vi "Module Loop.vi"(8 "error in (no error)":errorcluster, 11 "SoftVar Module in":refnum<class "SoftVar Module.lvclass">) -> (0 "error out":errorcluster, 3 "SoftVar Module out":refnum<class "SoftVar Module.lvclass">)   [LabVIEW 2023, in "Volatus.lvlib" / "SoftVar Module.lvclass"]
uses:
  SoftVar Module.lvclass
  SoftVar Module.lvclass/SoftVar Module.ctl
  Module/Module.lvclass
  messages/CmdAnalog/Data.ctl
  messages/CmdAnalog/CmdAnalog.lvlib
  lv-vecto/Vecto/Vecto.lvlib
  lv-vecto/Vecto/Group DBL/Group DBL.lvclass
  C:/dev/volatus/mts-volatus-super/libs/lv-volatus/Volatus/Module/Module.lvclass
  C:/dev/volatus/mts-volatus-super/libs/lv-volatus/Volatus/SoftVar Module/SoftVar Module.lvclass
panel:
  in  "Display":bool
  out "Values":T1(array[cluster])
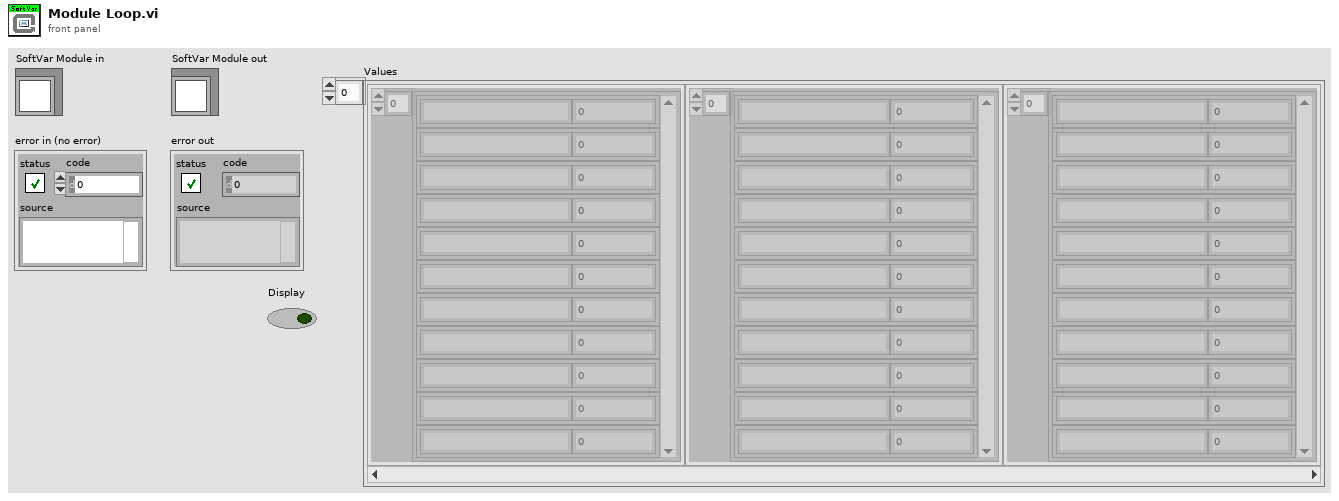
[diagram p1: front panel]
types:
  T1 = cluster{cluster{"Name":string, "Scaled":dbl}[]}[]
  T2 = enum32{"Invalid", "Standard", "Closed", "Hidden", "Minimized", "Maximized"}
  T3 = typedef "CmdAnalog.lvlib/Data.ctl" = cluster{"channel":string, "value":dbl}
  T4 = cluster{cluster{"String":string, "Scaled":dbl}[]}
  T5 = typedef "CmdAnalogMultiple.lvlib/Data.ctl" = cluster{"values":T3[]}
  T6 = typedef "CmdDigitalMultiple.lvlib/Data.ctl" = cluster{"values":T7[]}
  T7 = typedef "CmdDigital.lvlib/Data.ctl" = cluster{"channel":string, "value":bool}
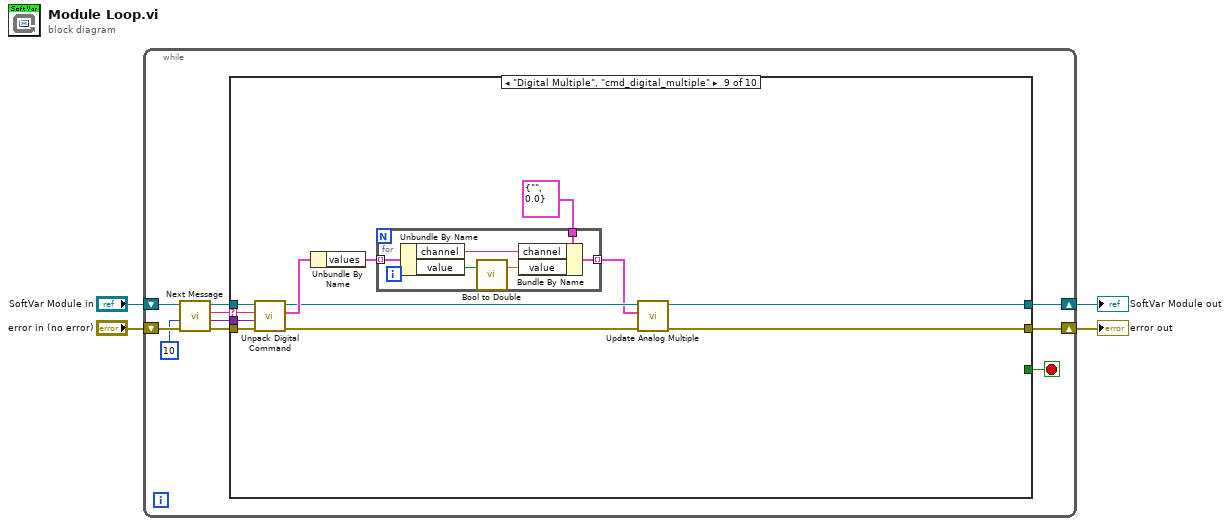
[diagram p0: block diagram]
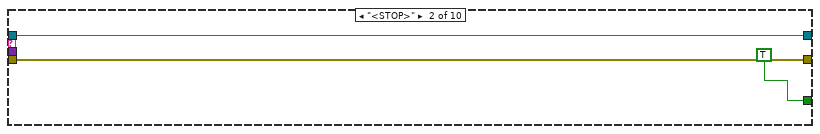
[diagram p3: hidden frame]
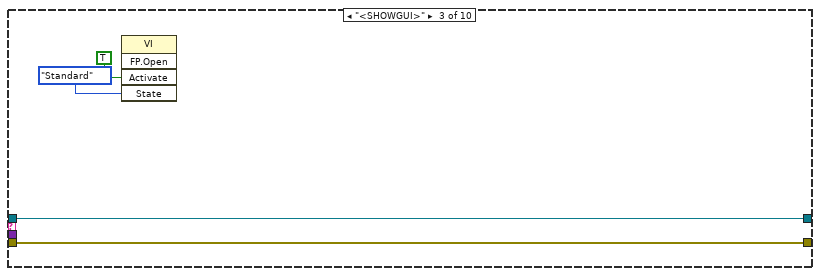
[diagram p4: hidden frame]
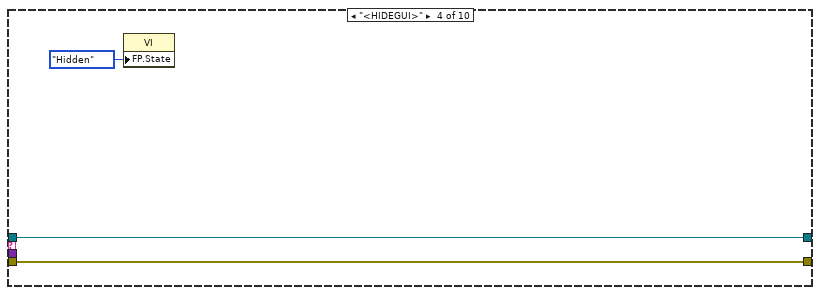
[diagram p5: hidden frame]
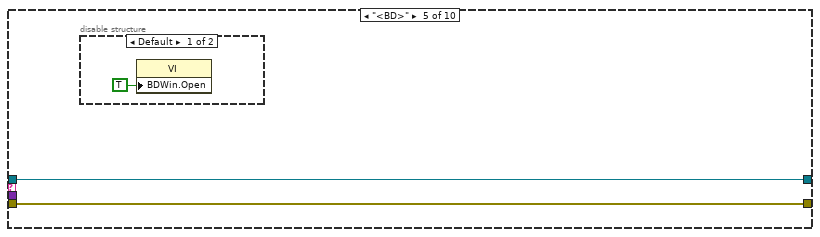
[diagram p6: hidden frame]
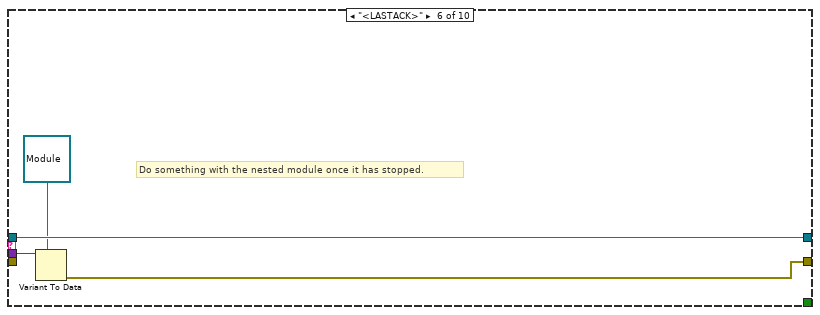
[diagram p8: hidden frame]
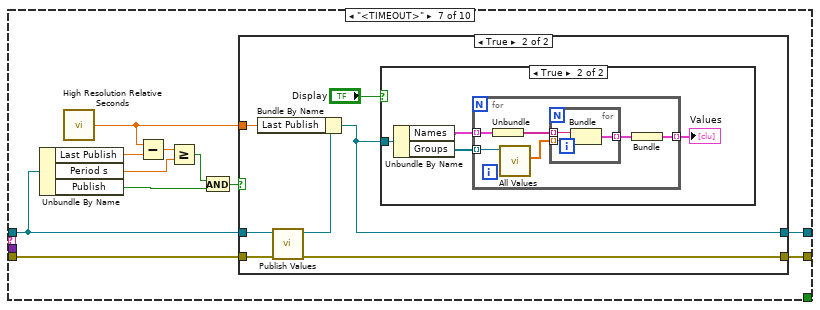
[diagram p9: hidden frame]
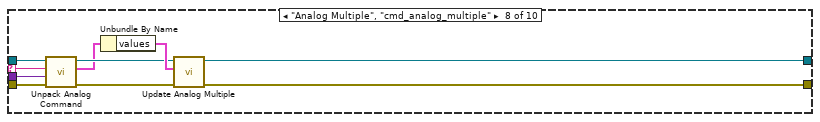
[diagram p12: hidden frame]
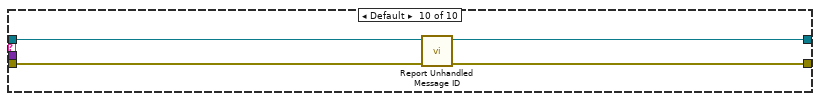
[diagram p13: hidden frame]
diagram:
  n1 = while {
    shift-right: [w9] -> w2
    shift-left: "SoftVar Module in" -> [w14]
    shift-right: [w8] -> w1
    shift-left: "error in (no error)" -> [w13]
    stop <- w7 stop-if-true
    n2 = call "Next Message.vi"("error in (no error)"=w13, "Timeout/Period ms (-1)"=10 ("Timeout ms (-1)"), "Module in"=w14) -> ("error out"=w12:errorcluster, "Data"=w6:variant, "ID"=w11:string, "Module out"=w10:refnum<class "SoftVar Module.lvclass">)  [unwired: 5 in]
    n3 = case shown="\"Digital Multiple\", \"cmd_digital_multiple\"" w11 {
      selector: w11 -> [_ _ _ _ _ _ _ w72 w84 _]
      tunnel: w12 -> [w15 w18 w22 w25 w27 _ w41 w70 w85 w98]
      tunnel: w10 -> [w16 w19 w23 w26 w28 w33 w42 w73 w86 w96]
      tunnel: [w16 w19 w23 w26 w28 w33 w34 w74 w78 w95] -> w9
      tunnel: [w15 w18 w22 w25 w27 w30 w35 w75 w77 w97] -> w8
      tunnel: [_ TRUE _ _ _ _ _ _ _ _] -> w7
      tunnel: w6 -> [_ _ _ _ _ w32 _ w71 w83 _]
      frame "<CLOSE>" {
      }
      frame "<STOP>" {
      }
      frame "<SHOWGUI>" {
        n4 = invoke class="VI" method="FP.Open"("Activate"=TRUE ("Activate?"), "State"=T2."Standard") -> ()  [unwired: 3 in, 5 out]
      }
      frame "<HIDEGUI>" {
        n5 = property class="VI"("FP.State"=T2."Hidden" ("Front Panel Window:State")) -> ()  [unwired: 2 in, 2 out]
      }
      frame "<BD>" {
        n6 = disable-structure shown="Default" {
          frame condition #0 (active) {
            n7 = property class="VI"("BDWin.Open"=TRUE ("Block Diagram Window:Open")) -> ()  [unwired: 2 in, 2 out]
          }
          frame condition #1 {
          }
        }
      }
      frame "<LASTACK>" {
        # "Do something with the nested module once it has stopped."
        n8 = Variant To Data(type=refnum<class "Module.lvclass"> refnum ("Volatus:Module"), Variant=w32) -> (error out=w30:errorcluster)  [unwired: 1 in, 1 out]
      }
      frame "<TIMEOUT>" {
        n9 = Unbundle By Name(w42) -> ("Last Publish"=w44:dbl, "Period s"=w38:dbl, "Publish"=w39:bool)
        n10 = call <vilib>:"High Resolution Relative Seconds.vi"() -> ("relative seconds"=w36:dbl)
        n11 = Subtract(x=w36, y=w44) -> (x-y=w43:dbl)
        n12 = Greater Or Equal?(x=w43, y=w38) -> (x >= y?=w40:bool)
        n13 = And(x=w40, y=w39) -> (x .and. y?=w37:bool)
        n14 = case shown="True" w37 {
          tunnel: w42 -> [w46 w53]
          tunnel: w41 -> [w45 w52]
          tunnel: w36 -> [_ w50]
          tunnel: [w45 w49] -> w35
          tunnel: [w46 w48] -> w34
          frame False {
          }
          frame True {
            n15 = call "Publish Values.vi"("error in (no error)"=w52, "SoftVar Module in"=w53) -> ("error out"=w49:errorcluster, "SoftVar Module out"=w51:refnum<class "SoftVar Module.lvclass">)  [unwired: 8 in]
            n16 = Bundle By Name(cluster=w51, "Last Publish"=w50) -> (w48:refnum<class "SoftVar Module.lvclass">)
            n17 = case shown="True" "Display" {
              tunnel: w48 -> [_ w57]
              frame False {
              }
              frame True {
                n18 = Unbundle By Name(w57) -> ("Names"=w54:cluster{"Names":string[]}[], "Groups"=w56:refnum<class "Group DBL.lvclass">[])
                n19 = for {
                  tunnel: w56 -> [w60] mode=indexing
                  tunnel: [w61] -> w55 mode=indexing
                  tunnel: w54 -> [w59] mode=indexing
                  n20 = Unbundle(w59) -> ("Names"=w58:string[])
                  n21 = call "All Values.vi"("Group in"=w60) -> ("Scaled"=w63:dbl[])  [unwired: 6 in, 4 out]
                  n22 = for {
                    tunnel: w58 -> [w66] mode=indexing
                    tunnel: w63 -> [w65] mode=indexing
                    tunnel: [w64] -> w62 mode=indexing
                    n23 = Bundle("String"=w66, "Scaled"=w65) -> (w64:cluster{"String":string, "Scaled":dbl})  [unwired: 1 in]
                  }
                  n24 = Bundle(w62) -> (w61:T4)  [unwired: 1 in]
                }
                "Values" <- w55
              }
            }
          }
        }
      }
      frame "Analog Multiple", "cmd_analog_multiple" {
        n25 = call "Unpack Analog Command.vi"("error in (no error)"=w70, "Data"=w71, "Type"=w72, "Module in"=w73) -> ("error out"=w69:errorcluster, "CmdAnalogMultiple"=w67:T5, "Module out"=w68:refnum<class "SoftVar Module.lvclass">)  [unwired: 3 in, 2 out]
        n26 = Unbundle By Name(w67) -> ("values"=w76:T3[])
        n27 = call "Update Analog Multiple.vi"("error in (no error)"=w69, "Channels"=w76, "SoftVar Module in"=w68) -> ("error out"=w75:errorcluster, "SoftVar Module out"=w74:refnum<class "SoftVar Module.lvclass">)  [unwired: 7 in]
      }
      frame "Digital Multiple", "cmd_digital_multiple" {
        n28 = call "Unpack Digital Command.vi"("error in (no error)"=w85, "Data"=w83, "Type"=w84, "Module in"=w86) -> ("error out"=w80:errorcluster, "CmdDigitalMultiple"=w82:T6, "Module out"=w81:refnum<class "SoftVar Module.lvclass">)  [unwired: 3 in, 2 out]
        n29 = Unbundle By Name(w82) -> ("values"=w88:T7[])
        n30 = for {
          tunnel: w88 -> [w94] mode=indexing
          tunnel: T3 {"channel"="", "value"=0.0} ("CmdAnalog") -> [w92]
          tunnel: [w89] -> w79 mode=indexing
          n31 = Unbundle By Name(w94) -> ("channel"=w91:string, "value"=w93:bool)
          n32 = call "Bool to Double.vi"("Bool"=w93) -> ("Double"=w90:dbl)  [unwired: 2 in]
          n33 = Bundle By Name(cluster=w92, "channel"=w91, "value"=w90) -> (w89:T3)
        }
        n34 = call "Update Analog Multiple.vi"("error in (no error)"=w80, "Channels"=w79, "SoftVar Module in"=w81) -> ("error out"=w77:errorcluster, "SoftVar Module out"=w78:refnum<class "SoftVar Module.lvclass">)  [unwired: 7 in]
      }
      frame Default {
        n35 = call "Report Unhandled Message ID.vi"("error in (no error)"=w98, "Module in"=w96) -> ("error out"=w97:errorcluster, "Module out"=w95:refnum<class "SoftVar Module.lvclass">)  [unwired: 8 in]
      }
    }
  }
  "error out" <- w1
  "SoftVar Module out" <- w2
